vi "Lab Panel V5.22.vi"() -> ()   [LabVIEW 2013] (continued)
                n1766 = property on="SET LAB01-2" class="Clust (strict)"("DisabledEnum"=w3311) -> ()  [unwired: 2 in, 2 out]
                n1767 = property on="SET LAB02-1" class="Clust (strict)"("DisabledEnum"=w3310) -> ()  [unwired: 2 in, 2 out]
                n1768 = property on="SET LAB02-2" class="Clust (strict)"("DisabledEnum"=w3309) -> ()  [unwired: 2 in, 2 out]
                n1769 = property on="SET LAB03-1" class="Clust (strict)"("DisabledEnum"=w3308) -> ()  [unwired: 2 in, 2 out]
                n1770 = property on="O/I  LAB01-1" class="Bool (strict)"("DisabledEnum"=w3312) -> ()  [unwired: 2 in, 2 out]
                n1771 = property on="O/I  LAB01-2" class="Bool (strict)"("DisabledEnum"=w3311) -> ()  [unwired: 2 in, 2 out]
                n1772 = property on="O/I  LAB02-1" class="Bool (strict)"("DisabledEnum"=w3310) -> ()  [unwired: 2 in, 2 out]
                n1773 = property on="O/I  LAB02-2" class="Bool (strict)"("DisabledEnum"=w3309) -> ()  [unwired: 2 in, 2 out]
                n1774 = property on="O/I  LAB03-1" class="Bool (strict)"("DisabledEnum"=w3308) -> ()  [unwired: 2 in, 2 out]
              }
              frame #1 {
                n1775 = Select(t=2, s=w3342, f=0) -> (s? t:f=w3333:i32)
                n1776 = Select(t=2, s=w3341, f=0) -> (s? t:f=w3334:i32)
                n1777 = Select(t=2, s=w3338, f=0) -> (s? t:f=w3337:i32)
                n1778 = Select(t=2, s=w3339, f=0) -> (s? t:f=w3336:i32)
                n1779 = Select(t=2, s=w3340, f=0) -> (s? t:f=w3335:i32)
                n1780 = property on="SELECT LAB05-2" class="RadioBtnsControl (strict)"("DisabledEnum"=w3333) -> ()  [unwired: 2 in, 2 out]
                n1781 = property on="SELECT LAB05-1" class="RadioBtnsControl (strict)"("DisabledEnum"=w3334) -> ()  [unwired: 2 in, 2 out]
                n1782 = property on="SELECT LAB03-2" class="RadioBtnsControl (strict)"("DisabledEnum"=w3337) -> ()  [unwired: 2 in, 2 out]
                n1783 = property on="SELECT LAB04-1" class="RadioBtnsControl (strict)"("DisabledEnum"=w3336) -> ()  [unwired: 2 in, 2 out]
                n1784 = property on="SELECT LAB04-2" class="RadioBtnsControl (strict)"("DisabledEnum"=w3335) -> ()  [unwired: 2 in, 2 out]
                n1785 = property on="SET LAB05-2" class="Clust (strict)"("DisabledEnum"=w3333) -> ()  [unwired: 2 in, 2 out]
                n1786 = property on="SET LAB05-1" class="Clust (strict)"("DisabledEnum"=w3334) -> ()  [unwired: 2 in, 2 out]
                n1787 = property on="SET LAB03-2" class="Clust (strict)"("DisabledEnum"=w3337) -> ()  [unwired: 2 in, 2 out]
                n1788 = property on="SET LAB04-1" class="Clust (strict)"("DisabledEnum"=w3336) -> ()  [unwired: 2 in, 2 out]
                n1789 = property on="SET LAB04-2" class="Clust (strict)"("DisabledEnum"=w3335) -> ()  [unwired: 2 in, 2 out]
                n1790 = property on="O/I  LAB05-2" class="Bool (strict)"("DisabledEnum"=w3333) -> ()  [unwired: 2 in, 2 out]
                n1791 = property on="O/I  LAB05-1" class="Bool (strict)"("DisabledEnum"=w3334) -> ()  [unwired: 2 in, 2 out]
                n1792 = property on="O/I  LAB04-1" class="Bool (strict)"("DisabledEnum"=w3336) -> ()  [unwired: 2 in, 2 out]
                n1793 = property on="O/I  LAB04-2" class="Bool (strict)"("DisabledEnum"=w3335) -> ()  [unwired: 2 in, 2 out]
                n1794 = property on="O/I  LAB03-2" class="Bool (strict)"("DisabledEnum"=w3337) -> ()  [unwired: 2 in, 2 out]
                n1795 = Not(x=w3342) -> (.not. x?=w3343:bool)
                n1796 = Not(x=w3341) -> (.not. x?=w3344:bool)
                n1797 = Not(x=w3340) -> (.not. x?=w3345:bool)
                n1798 = property on="RESULT LAB05-2" class="Bool (strict)"("Visible"=w3343) -> ()  [unwired: 2 in, 2 out]
                n1799 = property on="RESULT LAB05-1" class="Bool (strict)"("Visible"=w3344) -> ()  [unwired: 2 in, 2 out]
                n1800 = Not(x=w3339) -> (.not. x?=w3346:bool)
                n1801 = property on="RESULT LAB04-2" class="Bool (strict)"("Visible"=w3345) -> ()  [unwired: 2 in, 2 out]
                n1802 = Not(x=w3338) -> (.not. x?=w3347:bool)
                n1803 = property on="RESULT LAB04-1" class="Bool (strict)"("Visible"=w3346) -> ()  [unwired: 2 in, 2 out]
                n1804 = property on="RESULT LAB03-2" class="Bool (strict)"("Visible"=w3347) -> ()  [unwired: 2 in, 2 out]
              }
              frame #2 {
                # "disable calibrate if any test running"
                n1805 = Or(x=w3370, y=w3369) -> (x .or. y?=w3363:bool)
                n1806 = Or(x=w3372, y=w3371) -> (x .or. y?=w3365:bool)
                n1807 = Or(x=w3376, y=w3375) -> (x .or. y?=w3367:bool)
                n1808 = Or(x=w3374, y=w3373) -> (x .or. y?=w3366:bool)
                n1809 = Or(x=w3378, y=w3377) -> (x .or. y?=w3368:bool)
                n1810 = Or(x=w3366, y=w3365) -> (x .or. y?=w3364:bool)
                n1811 = Or(x=w3368, y=w3367) -> (x .or. y?=w3362:bool)
                n1812 = Or(x=w3364, y=w3363) -> (x .or. y?=w3361:bool)
                n1813 = Or(x=w3362, y=w3361) -> (x .or. y?=w3360:bool)
                n1814 = case shown="False" w3360 {
                  tunnel: [0 2] -> w3359
                  frame False {
                  }
                  frame True {
                  }
                }
                n1815 = property on="JIG TEST" class="Clust (strict)"("DisabledEnum"=w3359) -> ()  [unwired: 2 in, 2 out]
                n1816 = property on="Network Directory" class="Path"("DisabledEnum"=w3359) -> ()  [unwired: 2 in, 2 out]
                n1817 = property on="MAIL SETTINGS" class="Clust (strict)"("DisabledEnum"=w3359) -> ()  [unwired: 2 in, 2 out]
                n1818 = property on="SET (cal)" class="Bool (strict)"("DisabledEnum"=w3359) -> ()  [unwired: 2 in, 2 out]
                n1819 = property on="ADMIN" class="Bool (strict)"("DisabledEnum"=0) -> ()  [unwired: 2 in, 2 out]
              }
            }
          }
          frame #8 {
            # "drive jigs"
            n1820 = stacked-sequence {
              frame #0 {
                # "jig on"
                n1821 = local read "jig cycle"() -> (w3386:dbl)
                n1822 = property on="JIG TEST" class="Clust (strict)"() -> ("DisabledEnum"=w3383:T16)  [unwired: 2 in, 2 out]
                n1823 = Equal?(x=w3383, y=2) -> (x = y?=w3382:bool)
                n1824 = Equal?(x=w3386, y=0) -> (x = y?=w3384:bool)
                n1825 = And(x=w3384, y=w3382) -> (x .and. y?=w3381:bool)
                n1826 = case shown="True" w3381 {
                  frame False {
                  }
                  frame True {
                    n1827 = local read "run lab01-1"() -> (w3397:bool)
                    n1828 = local read "run lab01-2"() -> (w3396:bool)
                    n1829 = local read "run lab02-1"() -> (w3395:bool)
                    n1830 = local read "run lab02-2"() -> (w3394:bool)
                    n1831 = local read "run lab03-1"() -> (w3393:bool)
                    n1832 = local read "run lab03-2"() -> (w3392:bool)
                    n1833 = local read "run lab04-1"() -> (w3391:bool)
                    n1834 = local read "run lab04-2"() -> (w3390:bool)
                    n1835 = local read "run lab05-1"() -> (w3389:bool)
                    n1836 = local read "run lab05-2"() -> (w3388:bool)
                    n1837 = local write "JIG LAB03-2"(w3392) -> ()
                    n1838 = local write "JIG LAB01-1"(w3397) -> ()
                    n1839 = local write "JIG LAB01-2"(w3396) -> ()
                    n1840 = local write "JIG LAB02-1"(w3395) -> ()
                    n1841 = local write "JIG LAB02-2"(w3394) -> ()
                    n1842 = local write "JIG LAB03-1"(w3393) -> ()
                    n1843 = local write "JIG LAB04-1"(w3391) -> ()
                    n1844 = local write "JIG LAB04-2"(w3390) -> ()
                    n1845 = local write "JIG LAB05-1"(w3389) -> ()
                    n1846 = local write "JIG LAB05-2"(w3388) -> ()
                  }
                }
              }
              frame #1 {
                # "jig off"
                n1847 = local read "jig cycle"() -> (w3404:dbl)
                n1848 = local read "on loops"() -> (w3403:dbl)
                n1849 = property on="JIG TEST" class="Clust (strict)"() -> ("DisabledEnum"=w3402:T16)  [unwired: 2 in, 2 out]
                n1850 = Equal?(x=w3402, y=2) -> (x = y?=w3400:bool)
                n1851 = Equal?(x=w3404, y=w3403) -> (x = y?=w3399:bool)
                n1852 = And(x=w3399, y=w3400) -> (x .and. y?=w3398:bool)
                n1853 = case shown="True" w3398 {
                  frame False {
                  }
                  frame True {
                    w3455 = FALSE
                    w3456 = TRUE
                    w3454 = 2
                    n1854 = local read "SELECT LAB05-2"() -> (w3445:T3)
                    n1855 = local read "SELECT LAB04-2"() -> (w3447:T3)
                    n1856 = local read "SELECT LAB04-1"() -> (w3448:T3)
                    n1857 = local read "SELECT LAB05-1"() -> (w3446:T3)
                    n1858 = local read "SELECT LAB03-2"() -> (w3449:T3)
                    n1859 = local read "SELECT LAB02-1"() -> (w3452:T3)
                    n1860 = local read "SELECT LAB03-1"() -> (w3450:T3)
                    n1861 = local read "SELECT LAB02-2"() -> (w3451:T3)
                    n1862 = local read "SELECT LAB01-2"() -> (w3453:T3)
                    n1863 = local read "run lab05-1"() -> (w3415:bool)
                    n1864 = local read "run lab05-2"() -> (w3414:bool)
                    n1865 = local read "SELECT LAB01-1"() -> (w3457:T3)
                    n1866 = local read "run lab04-2"() -> (w3416:bool)
                    n1867 = local read "run lab04-1"() -> (w3417:bool)
                    n1868 = local read "run lab01-1"() -> (w3433:bool)
                    n1869 = local read "run lab01-2"() -> (w3422:bool)
                    n1870 = local read "run lab03-2"() -> (w3418:bool)
                    n1871 = local read "run lab03-1"() -> (w3419:bool)
                    n1872 = local read "run lab02-1"() -> (w3421:bool)
                    n1873 = local read "run lab02-2"() -> (w3420:bool)
                    n1874 = Equal?(x=w3454, y=w3450) -> (x = y?=w3428:bool)
                    n1875 = Equal?(x=w3454, y=w3449) -> (x = y?=w3427:bool)
                    n1876 = Equal?(x=w3454, y=w3448) -> (x = y?=w3426:bool)
                    n1877 = Equal?(x=w3454, y=w3447) -> (x = y?=w3425:bool)
                    n1878 = Equal?(x=w3454, y=w3446) -> (x = y?=w3424:bool)
                    n1879 = Equal?(x=w3454, y=w3445) -> (x = y?=w3423:bool)
                    n1880 = Equal?(x=w3454, y=w3457) -> (x = y?=w3434:bool)
                    n1881 = Equal?(x=w3454, y=w3452) -> (x = y?=w3430:bool)
                    n1882 = Equal?(x=w3454, y=w3451) -> (x = y?=w3429:bool)
                    n1883 = Equal?(x=w3454, y=w3453) -> (x = y?=w3431:bool)
                    n1884 = And(x=w3425, y=w3416) -> (x .and. y?=w3407:bool)
                    n1885 = And(x=w3428, y=w3419) -> (x .and. y?=w3410:bool)
                    n1886 = And(x=w3426, y=w3417) -> (x .and. y?=w3408:bool)
                    n1887 = And(x=w3423, y=w3414) -> (x .and. y?=w3405:bool)
                    n1888 = And(x=w3429, y=w3420) -> (x .and. y?=w3411:bool)
                    n1889 = And(x=w3427, y=w3418) -> (x .and. y?=w3409:bool)
                    n1890 = And(x=w3424, y=w3415) -> (x .and. y?=w3406:bool)
                    n1891 = And(x=w3431, y=w3422) -> (x .and. y?=w3413:bool)
                    n1892 = And(x=w3434, y=w3433) -> (x .and. y?=w3432:bool)
                    n1893 = And(x=w3430, y=w3421) -> (x .and. y?=w3412:bool)
                    n1894 = Select(t=w3456, s=w3432, f=w3455) -> (s? t:f=w3435:bool)
                    n1895 = Select(t=w3456, s=w3413, f=w3455) -> (s? t:f=w3436:bool)
                    n1896 = Select(t=w3456, s=w3412, f=w3455) -> (s? t:f=w3437:bool)
                    n1897 = Select(t=w3456, s=w3411, f=w3455) -> (s? t:f=w3438:bool)
                    n1898 = Select(t=w3456, s=w3410, f=w3455) -> (s? t:f=w3439:bool)
                    n1899 = Select(t=w3456, s=w3409, f=w3455) -> (s? t:f=w3440:bool)
                    n1900 = Select(t=w3456, s=w3408, f=w3455) -> (s? t:f=w3441:bool)
                    n1901 = Select(t=w3456, s=w3407, f=w3455) -> (s? t:f=w3442:bool)
                    n1902 = Select(t=w3456, s=w3406, f=w3455) -> (s? t:f=w3443:bool)
                    n1903 = Select(t=w3456, s=w3405, f=w3455) -> (s? t:f=w3444:bool)
                    n1904 = local write "JIG LAB03-2"(w3440) -> ()
                    n1905 = local write "JIG LAB02-1"(w3437) -> ()
                    n1906 = local write "JIG LAB02-2"(w3438) -> ()
                    n1907 = local write "JIG LAB01-2"(w3436) -> ()
                    n1908 = local write "JIG LAB03-1"(w3439) -> ()
                    n1909 = local write "JIG LAB01-1"(w3435) -> ()
                    n1910 = local write "JIG LAB05-2"(w3444) -> ()
                    n1911 = local write "JIG LAB04-1"(w3441) -> ()
                    n1912 = local write "JIG LAB05-1"(w3443) -> ()
                    n1913 = local write "JIG LAB04-2"(w3442) -> ()
                  }
                }
              }
            }
          }
          frame #9 {
            # "enable  jig test output if no test busy"
            n1914 = property on="JIG TEST" class="Clust (strict)"() -> ("DisabledEnum"=w3460:T16)  [unwired: 2 in, 2 out]
            n1915 = Equal?(x=w3460, y=0) -> (x = y?=w3458:bool)
            n1916 = case shown="True" w3458 {
              frame False {
              }
              frame True {
                n1917 = local read "JIG TEST"() -> (w3471:T10)
                n1918 = Unbundle(w3471) -> ("LAB01-1"=w3470:bool, "LAB01-2"=w3469:bool, "LAB02-1"=w3468:bool, "LAB02-2"=w3467:bool, "LAB03-1"=w3466:bool, "LAB03-2"=w3465:bool, "LAB04-1"=w3464:bool, "LAB04-2"=w3463:bool, "LAB05-1"=w3462:bool, "LAB05-2"=w3461:bool)
                n1919 = local write "JIG LAB05-1"(w3462) -> ()
                n1920 = local write "JIG LAB05-2"(w3461) -> ()
                n1921 = local write "JIG LAB04-1"(w3464) -> ()
                n1922 = local write "JIG LAB04-2"(w3463) -> ()
                n1923 = local write "JIG LAB03-2"(w3465) -> ()
                n1924 = local write "JIG LAB01-1"(w3470) -> ()
                n1925 = local write "JIG LAB02-1"(w3468) -> ()
                n1926 = local write "JIG LAB03-1"(w3466) -> ()
                n1927 = local write "JIG LAB01-2"(w3469) -> ()
                n1928 = local write "JIG LAB02-2"(w3467) -> ()
              }
            }
          }
          frame #10 {
            # "Drive digital output and reset USB and temperature network if required."
            n1929 = global read "Global display 3.vi" "cycle O/F"() -> (w3481:bool)
            n1930 = local read "O/I  LAB05-2"() -> (w3474:bool)
            n1931 = local read "O/I  LAB05-1"() -> (w3476:bool)
            n1932 = local read "JIG LAB05-2"() -> (w3473:bool)
            n1933 = local read "O/I  LAB04-2"() -> (w3478:bool)
            n1934 = local read "JIG LAB05-1"() -> (w3475:bool)
            n1935 = local read "JIG LAB04-2"() -> (w3477:bool)
            n1936 = local read "O/I  LAB03-1"() -> (w3492:bool)
            n1937 = local read "O/I  LAB04-1"() -> (w3488:bool)
            n1938 = local read "O/I  LAB02-1"() -> (w3496:bool)
            n1939 = local read "O/I  LAB02-2"() -> (w3494:bool)
            n1940 = local read "O/I  LAB03-2"() -> (w3490:bool)
            n1941 = local read "JIG LAB04-1"() -> (w3487:bool)
            n1942 = local read "JIG LAB03-2"() -> (w3489:bool)
            n1943 = local read "O/I  LAB01-2"() -> (w3498:bool)
            n1944 = local read "JIG LAB02-1"() -> (w3495:bool)
            n1945 = local read "JIG LAB02-2"() -> (w3493:bool)
            n1946 = local read "JIG LAB03-1"() -> (w3491:bool)
            n1947 = local read "O/I  LAB01-1"() -> (w3500:bool)
            n1948 = local read "JIG LAB01-2"() -> (w3497:bool)
            n1949 = local read "JIG LAB01-1"() -> (w3499:bool)
            n1950 = case shown="False" w3481 {
              tunnel: [w3598 FALSE] -> w3480
              frame False {
                n1951 = local read "Analog error"() -> (w3597:bool)
                n1952 = local read "Reset Measuring"() -> (w3596:bool)
                n1953 = Or(x=w3596, y=w3597) -> (x .or. y?=w3598:bool)
              }
              frame True {
              }
            }
            n1954 = Build Array(w3493, w3492, w3491, w3490, w3489, w3488, w3487) -> (w3485:bool[])
            n1955 = Build Array(w3500, w3499, w3498, w3497, w3496, w3495, w3494) -> (w3486:bool[])
            n1956 = Build Array(w3478, w3477, w3476, w3475, w3474, w3473, FALSE) -> (w3484:bool[])
            n1957 = Not(x=w3481) -> (.not. x?=w3482:bool)
            n1958 = local read "Simulate"() -> (w3483:bool)
            n1959 = And(x=w3482, y=w3480) -> (x .and. y?=w3479:bool)
            n1960 = stacked-sequence {
              tunnel: w3486 -> [w3504 w3510]
              tunnel: w3485 -> [w3503 w3509]
              tunnel: w3484 -> [w3502 w3508]
              tunnel: w3483 -> [w3501 w3511]
              tunnel: w3479 -> [_ w3512]
              frame #0 {
                # "drive outputs for normal use"
                n1961 = case shown="False" w3501 {
                  tunnel: w3504 -> [w3507 _]
                  tunnel: w3503 -> [w3506 _]
                  tunnel: w3502 -> [w3505 _]
                  frame False {
                    n1962 = call "sub vi - Drive Relays All v6.vi"("Array #2"=w3505, "Array #1"=w3506, "Array #0"=w3507) -> ()  [unwired: 8 in, 1 out]
                  }
                  frame True {
                  }
                }
              }
              frame #1 {
                # "USB  reset routine"
                n1963 = case shown="True" w3512 {
                  tunnel: w3511 -> [_ w3516]
                  tunnel: w3510 -> [_ w3515]
                  tunnel: w3509 -> [_ w3514]
                  tunnel: w3508 -> [_ w3513]
                  frame False {
                  }
                  frame True {
                    n1964 = stacked-sequence {
                      seq-local: [w3518 _ _ _] -> [_ w3524 _ _]
                      tunnel: w3516 -> [_ w3528 _ _]
                      tunnel: w3515 -> [_ w3527 _ _]
                      tunnel: w3514 -> [_ w3526 _ _]
                      tunnel: w3513 -> [_ w3525 _ _]
                      frame #0 {
                        n1965 = case shown="False" "Auto Reset" {
                          tunnel: [w3521 FALSE] -> w3519
                          frame False {
                            n1966 = Two Button Dialog(message="System reset") -> (T button?=w3521:bool)  [unwired: 2 in]
                          }
                          frame True {
                          }
                        }
                        n1967 = local write "Tab Control 2"(5) -> ()
                        n1968 = Or(x="Auto Reset", y=w3519) -> (x .or. y?=w3518:bool)
                      }
                      frame #1 {
                        n1969 = disable-structure shown="Disabled" {
                          disable-tunnel: w3528 -> [w3533 _]
                          disable-tunnel: w3527 -> [w3532 _]
                          disable-tunnel: w3526 -> [w3531 _]
                          disable-tunnel: w3525 -> [w3530 _]
                          disable-tunnel: w3524 -> [w3529 _]
                          frame Disabled {
                            n1970 = case shown="True" w3529 {
                              tunnel: w3533 -> [_ w3539]
                              tunnel: w3532 -> [_ w3538]
                              tunnel: w3531 -> [_ w3537]
                              tunnel: w3530 -> [_ w3536]
                              frame False {
                              }
                              frame True {
                                n1971 = stacked-sequence {
                                tunnel: w3539 -> [_ w3557 _]
                                tunnel: bool[] [] -> [w3542 w3556 w3566]
                                tunnel: w3538 -> [_ _ w3565]
                                tunnel: w3537 -> [w3541 _ w3564]
                                tunnel: w3536 -> [w3540 _ w3563]
                                tunnel: 3000 -> [w3543 _ w3562]
                                frame #0 {
                                # "switch off test stations for system reset"
                                n1972 = stacked-sequence {
                                tunnel: w3543 -> [w3547 w3551 w3553]
                                tunnel: w3542 -> [w3546 w3550 w3554]
                                tunnel: w3541 -> [w3545 _ _]
                                tunnel: w3540 -> [w3544 w3549 _]
                                frame #0 {
                                # "drive 1st 7 inputs"
                                n1973 = call "sub vi - Drive Relays All v6.vi"("Array #2"=w3544, "Array #1"=w3545, "Array #0"=w3546) -> ()  [unwired: 8 in, 1 out]
                                n1974 = call "Message Display V1.vi"("Message"="Delay off LAB 01-1 to 02-1", "Delay mS"=w3547) -> ()  [unwired: 10 in]
                                }
                                frame #1 {
                                # "drive 2nd 7 inputs"
                                n1975 = call "sub vi - Drive Relays All v6.vi"("Array #2"=w3549, "Array #1"=w3550, "Array #0"=w3550) -> ()  [unwired: 8 in, 1 out]
                                n1976 = call "Message Display V1.vi"("Message"="Delay off LAB 02-2 to 04-1", "Delay mS"=w3551) -> ()  [unwired: 10 in]
                                }
                                frame #2 {
                                # "drive 3rd 7 inputs"
                                n1977 = call "sub vi - Drive Relays All v6.vi"("Array #2"=w3554, "Array #1"=w3554, "Array #0"=w3554) -> ()  [unwired: 8 in, 1 out]
                                n1978 = call "Message Display V1.vi"("Message"="Delay off LAB 04-2 to 05-2", "Delay mS"=w3553) -> ()  [unwired: 10 in]
                                }
                                }
                                }
                                frame #1 {
                                # "reset all usb modules"
                                n1979 = stacked-sequence {
                                tunnel: w3557 -> [_ w3561]
                                tunnel: w3556 -> [w3559 _]
                                frame #0 {
                                n1980 = call "sub vi - Drive Relays All v6.vi"("Array #2"=bool[] [FALSE, FALSE, FALSE, FALSE, FALSE, FALSE, TRUE], "Array #1"=w3559, "Array #0"=w3559) -> ()  [unwired: 8 in, 1 out]
                                }
                                frame #1 {
                                n1981 = call "Reset Meas v 4.vi"("simulate"=w3561) -> ("Reset Error"=→"Reset Error":bool)  [unwired: 10 in]
                                }
                                }
                                }
                                frame #2 {
                                # "switch test stations back on after reset"
                                n1982 = stacked-sequence {
                                tunnel: w3566 -> [w3570 w3573 _]
                                tunnel: w3565 -> [w3569 w3575 w3580]
                                tunnel: w3562 -> [w3568 w3571 w3577]
                                tunnel: w3564 -> [_ w3574 w3579]
                                tunnel: w3563 -> [_ _ w3576]
                                frame #0 {
                                # "drive 1st 7 inputs"
                                n1983 = call "sub vi - Drive Relays All v6.vi"("Array #2"=w3570, "Array #1"=w3570, "Array #0"=w3569) -> ()  [unwired: 8 in, 1 out]
                                n1984 = call "Message Display V1.vi"("Message"="Delay on LAB 01-1 to 02-1", "Delay mS"=w3568) -> ()  [unwired: 10 in]
                                }
                                frame #1 {
                                # "drive 1st & 2nd outputs"
                                n1985 = call "sub vi - Drive Relays All v6.vi"("Array #2"=w3573, "Array #1"=w3574, "Array #0"=w3575) -> ()  [unwired: 8 in, 1 out]
                                n1986 = call "Message Display V1.vi"("Message"="Delay on LAB 02-2 to 04-1", "Delay mS"=w3571) -> ()  [unwired: 10 in]
                                }
                                frame #2 {
                                n1987 = call "sub vi - Drive Relays All v6.vi"("Array #2"=w3576, "Array #1"=w3579, "Array #0"=w3580) -> ()  [unwired: 8 in, 1 out]
                                n1988 = call "Message Display V1.vi"("Message"="Delay on LAB 04-2 to 05-2", "Delay mS"=w3577) -> ()  [unwired: 10 in]
                                }
                                }
                                }
                                }
                              }
                            }
                          }
                          frame Enabled {
                          }
                        }
                      }
                      frame #2 {
                        w3585 = 0
                        w3586 = FALSE
                        # "set all back to zero"
                        n1989 = local read "Total USB resets"() -> (w3582:dbl)
                        n1990 = local read "Resets Done"() -> (w3584:dbl)
                        n1991 = local write "Reset Measuring"(w3586) -> ()
                        n1992 = local write "Analog error"(w3586) -> ()
                        n1993 = local write "Error USB #0"(w3586) -> ()
                        n1994 = local write "Error USB #1"(w3586) -> ()
                        n1995 = local write "Error USB #2"(w3586) -> ()
                        n1996 = local write "Er USB#0"(w3585) -> ()
                        n1997 = local write "Er USB#1"(w3585) -> ()
                        n1998 = local write "Er USB#2"(w3585) -> ()
                        n1999 = Increment(x=w3582) -> (x+1=w3581:dbl)
                        n2000 = Increment(x=w3584) -> (x+1=→"Resets Done":dbl)
                        n2001 = local write "Total USB resets"(w3581) -> ()
                      }
                      frame #3 {
                        # "mail reset value"
                        n2002 = disable-structure shown="Disabled" {
                          frame Disabled {
                            n2003 = local read "Total USB resets"() -> (w3592:dbl)
                            n2004 = local read "MAIL SETTINGS"() -> (w3588:T7)
                            n2005 = local read "Mail Test File To:"() -> (w3593:string)
                            n2006 = Number To Decimal String(number=w3592) -> (decimal integer string=w3590:string)  [unwired: 1 in]
                            n2007 = Unbundle(w3588) -> ("OUT SERVER ADDRESS"=w3595:string, "FROM ACCOUNT"=w3594:string)  [unwired: 5 out]
                            n2008 = Concatenate Strings("Total USB resets: ", w3590) -> (w3589:string)
                            n2009 = call "sub vi - send mail v5.vi"("TO:"=w3593, "subject"=w3589, "from"=w3594, "out going server"=w3595) -> ("error out"=w3587:errorcluster)  [unwired: 11 in]
                            n2010 = Bundle(cluster=w3588, "mail error"=w3587) -> ()  [unwired: 6 in, 1 out]
                          }
                          frame Enabled {
                          }
                        }
                      }
                    }
                  }
                }
              }
            }
          }
          frame #11 {
            # "get all analog values from USB devices"
            n2011 = local read "on loops"() -> (w3606:dbl)
            n2012 = local read "jig cycle"() -> (w3603:dbl)
            n2013 = Add(x=w3606, y=1) -> (x+y=w3604:dbl)
            n2014 = Equal?(x=w3603, y=1) -> (x = y?=w3600:bool)
            n2015 = Equal?(x=w3603, y=w3604) -> (x = y?=w3602:bool)
            n2016 = Or(x=w3600, y=w3602) -> (x .or. y?=w3601:bool)
            n2017 = global write "Global display 3.vi" "cycle O/F"(w3600) -> ()
            n2018 = case shown="True" w3601 {
              tunnel: w3600 -> [_ w3610]
              frame False {
              }
              frame True {
                n2019 = local read "Simulate"() -> (w3613:bool)
                n2020 = case shown="False" w3613 {
                  tunnel: [w3629 0.3 ("Analog loop time")] -> w3620
                  tunnel: [w3628 dynamicdata[] [] ("array GRAPH")] -> w3619
                  tunnel: [w3627 w3634] -> w3618
                  tunnel: [w3626 w3634] -> w3617
                  tunnel: [w3625 w3634] -> w3616
                  tunnel: [w3624 w3634] -> w3615
                  tunnel: [w3623 w3634] -> w3614
                  tunnel: w3610 -> [_ w3638]
                  tunnel: [w3622 "Ambient Volts"] -> w3609
                  tunnel: [w3621 bool[] []] -> w3608
                  frame False {
                    n2021 = call "sub vi - Read Analog All v9.3.vi"() -> ("Analog loop time"=w3629:dbl, "array GRAPH"=w3628:dynamicdata[], "LAB01"=w3627:T26, "LAB02"=w3626:T27, "LAB03"=w3625:T28, "LAB04"=w3624:T29, "deg C"=w3622:dbl, "USB Error"=w3621:bool[], "LAB05"=w3623:T30)  [unwired: 7 in]
                  }
                  frame True {
                    n2022 = local read "ON amps"() -> (w3632:dbl)
                    n2023 = local read "OFF amps"() -> (w3633:dbl)
                    n2024 = local read "VOLTS"() -> (w3636:dbl)
                    n2025 = local read "PF"() -> (w3635:dbl)
                    n2026 = Select(t=w3632, s=w3638, f=w3633) -> (s? t:f=w3637:dbl)
                    n2027 = Bundle("OFF amps"=w3637, "VOLTS"=w3636, "PF"=w3635, "OFF amps"=w3637, "VOLTS"=w3636, "PF"=w3635) -> (w3634:T31)  [unwired: 1 in]
                  }
                }
                n2028 = local read "Simulate"() -> (w3612:bool)
                n2029 = stacked-sequence {
                  seq-local: [w3643 _ _ _ _ _ _ _] -> [_ _ _ _ _ _ _ _]
                  seq-local: [w3642 _ _ _ _ _ _ _] -> [_ _ _ _ _ _ _ _]
                  seq-local: [w3641 _ _ _ _ _ _ _] -> [_ _ _ _ _ _ _ w3838]
                  tunnel: w3620 -> [_ w3696 _ _ _ _ _ _]
                  tunnel: w3619 -> [_ w3693 _ _ _ _ _ _]
                  tunnel: w3618 -> [_ _ w3723 _ _ _ _ _]
                  tunnel: w3617 -> [_ _ _ w3751 _ _ _ _]
                  tunnel: w3616 -> [_ _ _ _ w3779 _ _ _]
                  tunnel: w3615 -> [_ _ _ _ _ w3807 _ _]
                  tunnel: w3614 -> [_ _ _ _ _ _ w3835 _]
                  tunnel: w3612 -> [_ _ w3722 w3750 w3778 w3806 w3834 w3840]
                  tunnel: T14 {"1  (A) cal"=1.0, "1 (V) cal"=1.0, "1 (PF) cal"=1.0, "1 (TL) cal"=1.0, "1 (TN) cal"=1.0, "2 (A) cal"=1.0, "2 (V) cal"=1.0, "2 (PF) cal"=1.0, "2 (TL) cal"=1.0, "2 (TN) cal"=1.0} ("CAL LAB01") -> [_ _ w3721 w3749 w3777 w3805 w3833 _]
                  tunnel: w3609 -> [_ _ _ _ _ _ _ w3839]
                  tunnel: w3608 -> [w3646 _ _ _ _ _ _ _]
                  frame #0 {
                    n2030 = Index Array(array=w3646, index=2) -> (element=w3641:bool)
                    n2031 = Index Array(array=w3646, index=1) -> (element=w3642:bool)
                    n2032 = Index Array(array=w3646, index=0) -> (element=w3643:bool)
                    n2033 = local write "Error USB #2"(w3641) -> ()
                    n2034 = local write "Error USB #0"(w3643) -> ()
                    n2035 = local write "Error USB #1"(w3642) -> ()
                    n2036 = stacked-sequence {
                      tunnel: w3643 -> [w3650 _ _ _]
                      tunnel: w3642 -> [_ w3655 _ _]
                      tunnel: 0 -> [w3649 w3654 w3659 _]
                      tunnel: w3641 -> [_ _ w3660 _]
                      frame #0 {
                        n2037 = case shown="True" w3650 {
                          tunnel: w3649 -> [w3651 _]
                          frame False {
                            n2038 = local write "Er USB#0"(w3651) -> ()
                          }
                          frame True {
                            n2039 = local read "Er USB#0"() -> (w3653:dbl)
                            n2040 = Increment(x=w3653) -> (x+1=→"Er USB#0":dbl)
                          }
                        }
                      }
                      frame #1 {
                        n2041 = case shown="True" w3655 {
                          tunnel: w3654 -> [w3656 _]
                          frame False {
                            n2042 = local write "Er USB#1"(w3656) -> ()
                          }
                          frame True {
                            n2043 = local read "Er USB#1"() -> (w3658:dbl)
                            n2044 = Increment(x=w3658) -> (x+1=→"Er USB#1":dbl)
                          }
                        }
                      }
                      frame #2 {
                        n2045 = case shown="True" w3660 {
                          tunnel: w3659 -> [w3661 _]
                          frame False {
                            n2046 = local write "Er USB#2"(w3661) -> ()
                          }
                          frame True {
                            n2047 = local read "Er USB#2"() -> (w3663:dbl)
                            n2048 = Increment(x=w3663) -> (x+1=→"Er USB#2":dbl)
                          }
                        }
                      }
                      frame #3 {
                        w3669 = 5
                        n2049 = local read "Er USB#2"() -> (w3670:dbl)
                        n2050 = local read "Er USB#0"() -> (w3672:dbl)
                        n2051 = local read "Er USB#1"() -> (w3671:dbl)
                        n2052 = Greater Or Equal?(x=w3672, y=w3669) -> (x >= y?=w3667:bool)
                        n2053 = Greater Or Equal?(x=w3671, y=w3669) -> (x >= y?=w3666:bool)
                        n2054 = Greater Or Equal?(x=w3670, y=w3669) -> (x >= y?=w3665:bool)
                        n2055 = Or(x=w3667, y=w3666) -> (x .or. y?=w3668:bool)
                        n2056 = Or(x=w3668, y=w3665) -> (x .or. y?=→"Analog error":bool)
                      }
                    }
                  }
                  frame #1 {
                    # "display graph data on ADM page"
                    n2057 = local write "AI"(TRUE) -> ()
                    n2058 = global write "Global 1.vi" "RATE(Hz)"("RATE (Hz)") -> ()
                    n2059 = global write "Global 1.vi" "SAMPLES"("SAMPLES") -> ()
                    n2060 = Index Array(array=w3693, index=6) -> (element=→"LAB04-1 (GRAPH)":dynamicdata)
                    n2061 = Index Array(array=w3693, index=7) -> (element=→"LAB04-2 (GRAPH)":dynamicdata)
                    n2062 = Index Array(array=w3693, index=9) -> (element=→"LAB05-2 (GRAPH)":dynamicdata)
                    n2063 = Index Array(array=w3693, index=8) -> (element=→"LAB05-1 (GRAPH)":dynamicdata)
                    n2064 = Index Array(array=w3693, index=5) -> (element=→"LAB03-2 (GRAPH)":dynamicdata)
                    n2065 = Index Array(array=w3693, index=0) -> (element=→"LAB01-1 (GRAPH)":dynamicdata)
                    n2066 = Index Array(array=w3693, index=1) -> (element=→"LAB01-2 (GRAPH)":dynamicdata)
                    n2067 = Index Array(array=w3693, index=2) -> (element=→"LAB02-1 (GRAPH)":dynamicdata)
                    n2068 = Index Array(array=w3693, index=3) -> (element=→"LAB02-2 (GRAPH)":dynamicdata)
                    n2069 = Index Array(array=w3693, index=4) -> (element=→"LAB03-1 (GRAPH)":dynamicdata)
                    "AI loop time" <- w3696
                  }
                  frame #2 {
                    n2070 = case shown="False" w3722 {
                      tunnel: [w3724 w3725] -> w3720
                      tunnel: w3721 -> [_ w3725]
                      frame False {
                        n2071 = local read "CAL LAB01"() -> (w3724:T14)
                      }
                      frame True {
                      }
                    }
                    n2072 = Unbundle By Name(w3723) -> ("OFF amps"=w3719:dbl, "VOLTS"=w3718:dbl, "PF"=w3717:dbl, "OFF amps"=w3716:dbl, "VOLTS"=w3715:dbl, "PF"=w3714:dbl)
                    n2073 = Unbundle By Name(w3720) -> ("1  (A) cal"=w3713:dbl, "1 (V) cal"=w3712:dbl, "1 (PF) cal"=w3711:dbl, "2 (A) cal"=w3710:dbl, "2 (V) cal"=w3709:dbl, "2 (PF) cal"=w3708:dbl)  [unwired: 4 out]
                    n2074 = Multiply(x=w3719, y=w3713) -> (x*y=w3706:dbl)
                    n2075 = Multiply(x=w3718, y=w3712) -> (x*y=w3705:dbl)
                    n2076 = Multiply(x=w3717, y=w3711) -> (x*y=w3704:dbl)
                    n2077 = Multiply(x=w3716, y=w3710) -> (x*y=w3702:dbl)
                    n2078 = Multiply(x=w3715, y=w3709) -> (x*y=w3701:dbl)
                    n2079 = Multiply(x=w3714, y=w3708) -> (x*y=w3700:dbl)
                    n2080 = local read "SIG LAB01-1"() -> (w3707:T2)
                    n2081 = local read "SIG LAB01-2"() -> (w3703:T2)
                    n2082 = Bundle By Name(cluster=w3707, "AMPS"=w3706, "VOLTS"=w3705, "PF"=w3704) -> (w3699:T2)
                    n2083 = Bundle By Name(cluster=w3703, "AMPS"=w3702, "VOLTS"=w3701, "PF"=w3700) -> (w3698:T2)
                    n2084 = global write "Global display 1.vi" "SIG LAB01-2"(w3698) -> ()
                    n2085 = global write "Global display 1.vi" "SIG LAB01-1"(w3699) -> ()
                    n2086 = local write "SIG LAB01-2"(w3698) -> ()
                    n2087 = local write "SIG LAB01-1"(w3699) -> ()
                  }
                  frame #3 {
                    n2088 = Unbundle By Name(w3751) -> ("OFF amps"=w3747:dbl, "VOLTS"=w3746:dbl, "PF"=w3745:dbl, "OFF amps"=w3744:dbl, "VOLTS"=w3743:dbl, "PF"=w3742:dbl)
                    n2089 = case shown="True" w3750 {
                      tunnel: [w3752 w3753] -> w3748
                      tunnel: w3749 -> [_ w3753]
                      frame False {
                        n2090 = local read "CAL LAB02"() -> (w3752:T15)
                      }
                      frame True {
                      }
                    }
                    n2091 = Unbundle By Name(w3748) -> ("1  (A) cal"=w3741:dbl, "1 (V) cal"=w3740:dbl, "1 (PF) cal"=w3739:dbl, "2 (A) cal"=w3738:dbl, "2 (V) cal"=w3737:dbl, "2 (PF) cal"=w3736:dbl)  [unwired: 4 out]
                    n2092 = Multiply(x=w3747, y=w3741) -> (x*y=w3734:dbl)
                    n2093 = Multiply(x=w3746, y=w3740) -> (x*y=w3733:dbl)
                    n2094 = Multiply(x=w3745, y=w3739) -> (x*y=w3732:dbl)
                    n2095 = Multiply(x=w3744, y=w3738) -> (x*y=w3730:dbl)
                    n2096 = Multiply(x=w3743, y=w3737) -> (x*y=w3729:dbl)
                    n2097 = Multiply(x=w3742, y=w3736) -> (x*y=w3728:dbl)
                    n2098 = local read "SIG LAB02-1"() -> (w3735:T2)
                    n2099 = local read "SIG LAB02-2"() -> (w3731:T2)
                    n2100 = Bundle By Name(cluster=w3735, "AMPS"=w3734, "VOLTS"=w3733, "PF"=w3732) -> (w3727:T2)
                    n2101 = Bundle By Name(cluster=w3731, "AMPS"=w3730, "VOLTS"=w3729, "PF"=w3728) -> (w3726:T2)
                    n2102 = global write "Global display 1.vi" "SIG LAB02-1"(w3727) -> ()
                    n2103 = local write "SIG LAB02-2"(w3726) -> ()
                    n2104 = global write "Global display 1.vi" "SIG LAB02-2"(w3726) -> ()
                    n2105 = local write "SIG LAB02-1"(w3727) -> ()
                  }
                  frame #4 {
                    n2106 = Unbundle By Name(w3779) -> ("OFF amps"=w3775:dbl, "VOLTS"=w3774:dbl, "PF"=w3773:dbl, "OFF amps"=w3772:dbl, "VOLTS"=w3771:dbl, "PF"=w3770:dbl)
                    n2107 = case shown="True" w3778 {
                      tunnel: [w3780 w3781] -> w3776
                      tunnel: w3777 -> [_ w3781]
                      frame False {
                        n2108 = local read "CAL LAB03"() -> (w3780:T14)
                      }
                      frame True {
                      }
                    }
                    n2109 = Unbundle By Name(w3776) -> ("1  (A) cal"=w3769:dbl, "1 (V) cal"=w3768:dbl, "1 (PF) cal"=w3767:dbl, "2 (A) cal"=w3766:dbl, "2 (V) cal"=w3765:dbl, "2 (PF) cal"=w3764:dbl)  [unwired: 4 out]
                    n2110 = Multiply(x=w3775, y=w3769) -> (x*y=w3762:dbl)
                    n2111 = Multiply(x=w3774, y=w3768) -> (x*y=w3756:dbl)
                    n2112 = Multiply(x=w3773, y=w3767) -> (x*y=w3761:dbl)
                    n2113 = Multiply(x=w3772, y=w3766) -> (x*y=w3759:dbl)
                    n2114 = Multiply(x=w3771, y=w3765) -> (x*y=w3758:dbl)
                    n2115 = Multiply(x=w3770, y=w3764) -> (x*y=w3757:dbl)
                    n2116 = local read "SIG LAB03-1"() -> (w3763:T2)
                    n2117 = local read "SIG LAB03-2"() -> (w3760:T2)
                    n2118 = Bundle By Name(cluster=w3763, "AMPS"=w3762, "VOLTS"=w3756, "PF"=w3761) -> (w3755:T2)
                    n2119 = Bundle By Name(cluster=w3760, "AMPS"=w3759, "VOLTS"=w3758, "PF"=w3757) -> (w3754:T2)
                    n2120 = global write "Global display 1.vi" "SIG LAB03-1"(w3755) -> ()
                    n2121 = global write "Global display 1.vi" "SIG LAB03-2"(w3754) -> ()
                    n2122 = local write "SIG LAB03-2"(w3754) -> ()
                    n2123 = local write "SIG LAB03-1"(w3755) -> ()
                  }
                  frame #5 {
                    n2124 = case shown="False" w3806 {
                      tunnel: [w3808 w3809] -> w3804
                      tunnel: w3805 -> [_ w3809]
                      frame False {
                        n2125 = local read "CAL LAB04"() -> (w3808:T14)
                      }
                      frame True {
                      }
                    }
                    n2126 = Unbundle By Name(w3807) -> ("OFF amps"=w3803:dbl, "VOLTS"=w3802:dbl, "PF"=w3801:dbl, "OFF amps"=w3800:dbl, "VOLTS"=w3799:dbl, "PF"=w3798:dbl)
                    n2127 = Unbundle By Name(w3804) -> ("1  (A) cal"=w3797:dbl, "1 (V) cal"=w3796:dbl, "1 (PF) cal"=w3795:dbl, "2 (A) cal"=w3794:dbl, "2 (V) cal"=w3793:dbl, "2 (PF) cal"=w3792:dbl)  [unwired: 4 out]
                    n2128 = Multiply(x=w3803, y=w3797) -> (x*y=w3790:dbl)
                    n2129 = Multiply(x=w3802, y=w3796) -> (x*y=w3789:dbl)
                    n2130 = Multiply(x=w3801, y=w3795) -> (x*y=w3788:dbl)
                    n2131 = Multiply(x=w3800, y=w3794) -> (x*y=w3786:dbl)
                    n2132 = Multiply(x=w3799, y=w3793) -> (x*y=w3785:dbl)
                    n2133 = Multiply(x=w3798, y=w3792) -> (x*y=w3784:dbl)
                    n2134 = local read "SIG LAB04-1"() -> (w3791:T2)
                    n2135 = local read "SIG LAB04-2"() -> (w3787:T2)
                    n2136 = Bundle By Name(cluster=w3791, "AMPS"=w3790, "VOLTS"=w3789, "PF"=w3788) -> (w3783:T2)
                    n2137 = Bundle By Name(cluster=w3787, "AMPS"=w3786, "VOLTS"=w3785, "PF"=w3784) -> (w3782:T2)
                    n2138 = global write "Global display 1.vi" "SIG LAB04-2"(w3782) -> ()
                    n2139 = global write "Global display 1.vi" "SIG LAB04-1"(w3783) -> ()
                    n2140 = local write "SIG LAB04-2"(w3782) -> ()
                    n2141 = local write "SIG LAB04-1"(w3783) -> ()
                  }
                  frame #6 {
                    n2142 = Unbundle By Name(w3835) -> ("OFF amps"=w3831:dbl, "VOLTS"=w3812:dbl, "PF"=w3830:dbl, "OFF amps"=w3829:dbl, "VOLTS"=w3828:dbl, "PF"=w3827:dbl)
                    n2143 = case shown="False" w3834 {
                      tunnel: [w3836 w3837] -> w3832
                      tunnel: w3833 -> [_ w3837]
                      frame False {
                        n2144 = local read "CAL LAB05"() -> (w3836:T14)
                      }
                      frame True {
                      }
                    }
                    n2145 = Unbundle By Name(w3832) -> ("1  (A) cal"=w3826:dbl, "1 (V) cal"=w3825:dbl, "1 (PF) cal"=w3824:dbl, "2 (A) cal"=w3823:dbl, "2 (V) cal"=w3822:dbl, "2 (PF) cal"=w3821:dbl)  [unwired: 4 out]
                    n2146 = Multiply(x=w3831, y=w3826) -> (x*y=w3819:dbl)
                    n2147 = Multiply(x=w3812, y=w3825) -> (x*y=w3818:dbl)
                    n2148 = Multiply(x=w3830, y=w3824) -> (x*y=w3817:dbl)
                    n2149 = Multiply(x=w3829, y=w3823) -> (x*y=w3815:dbl)
                    n2150 = Multiply(x=w3828, y=w3822) -> (x*y=w3814:dbl)
                    n2151 = Multiply(x=w3827, y=w3821) -> (x*y=w3813:dbl)
                    n2152 = local read "SIG LAB05-1"() -> (w3820:T2)
                    n2153 = local read "SIG LAB05-2"() -> (w3816:T2)
                    n2154 = Bundle By Name(cluster=w3820, "AMPS"=w3819, "VOLTS"=w3818, "PF"=w3817) -> (w3811:T2)
                    n2155 = Bundle By Name(cluster=w3816, "AMPS"=w3815, "VOLTS"=w3814, "PF"=w3813) -> (w3810:T2)
                    n2156 = global write "Global display 1.vi" "SIG LAB05-1"(w3811) -> ()
                    n2157 = global write "Global display 1.vi" "SIG LAB05-2"(w3810) -> ()
                    n2158 = local write "SIG LAB05-2"(w3810) -> ()
                    n2159 = local write "SIG LAB05-1"(w3811) -> ()
                  }
                  frame #7 {
                    n2160 = case shown="False" w3838 {
                      tunnel: w3840 -> [w3842 _]
                      tunnel: w3839 -> [w3841 _]
                      frame False {
                        # "update ambient referance temperature"
                        n2161 = case shown="True" w3842 {
                          tunnel: [w3845 100.0] -> w3844
                          frame False {
                            n2162 = local read "TEMP REF cal"() -> (w3845:dbl)
                          }
                          frame True {
                          }
                        }
                        n2163 = local read "Panel #"() -> (w3843:dbl)
                        n2164 = case shown="1" w3843 {
                          tunnel: w3844 -> [_ w3851]
                          tunnel: w3841 -> [_ w3850]
                          frame 0, Default {
                          }
                          frame 1 {
                            n2165 = Multiply(x=w3851, y=w3850) -> (x*y=w3849:dbl)
                            n2166 = Subtract(x=w3849, y=272) -> (x-y=w3847:dbl)
                            "Amb Tp" <- w3847
                            n2167 = local write "Ref deg C"(w3847) -> ()
                          }
                        }
                        "deg C (volts)" <- w3841
                      }
                      frame True {
                      }
                    }
                  }
                }
              }
            }
          }
          frame #12 {
            # "save test data to file"
            n2168 = Get Date/Time In Seconds() -> (seconds since 1Jan1904=w3852:timestamp)
            "File Time Stamp" <- w3852
            n2169 = local read "on loops"() -> (w3871:dbl)
            n2170 = local read "jig cycle"() -> (w3868:dbl)
            n2171 = Format Date/Time String(time format string (%c)="%H:%M%:%S", seconds (now)=w3852) -> (date/time string=w3856:string)  [unwired: 1 in]
            n2172 = Add(x=w3871, y=2) -> (x+y=w3869:dbl)
            n2173 = Build Array(w3856) -> (w3855:string[])
            n2174 = Equal?(x=w3868, y=1) -> (x = y?=w3854:bool)
            n2175 = Equal?(x=w3868, y=w3869) -> (x = y?=w3853:bool)
            n2176 = stacked-sequence {
              tunnel: w3867 -> [w3877 _ _ _ _ _ _ _ _ _]
              tunnel: w3866 -> [_ w3953 _ _ _ _ _ _ _ _]
              tunnel: w3865 -> [_ _ w4033 _ _ _ _ _ _ _]
              tunnel: w3864 -> [_ _ _ w4113 _ _ _ _ _ _]
              tunnel: w3863 -> [_ _ _ _ w4193 _ _ _ _ _]
              tunnel: w3862 -> [_ _ _ _ _ w4273 _ _ _ _]
              tunnel: w3861 -> [_ _ _ _ _ _ w4353 _ _ _]
              tunnel: w3860 -> [_ _ _ _ _ _ _ w4433 _ _]
              tunnel: w3859 -> [_ _ _ _ _ _ _ _ w4513 _]
              tunnel: w3858 -> [_ _ _ _ _ _ _ _ _ w4593]
              tunnel: w3855 -> [w3876 w3957 w4037 w4117 w4197 w4277 w4357 w4437 w4517 w4597]
              tunnel: w3854 -> [w3875 w3956 w4036 w4116 w4196 w4276 w4356 w4436 w4516 w4596]
              tunnel: w3853 -> [w3874 w3955 w4035 w4115 w4195 w4275 w4355 w4435 w4515 w4595]
              tunnel: w3852 -> [w3873 w3954 w4034 w4114 w4194 w4274 w4354 w4434 w4514 w4594]
              frame #0 {
                n2177 = case shown="True" w3877 {
                  tunnel: w3876 -> [_ w3882]
                  tunnel: w3875 -> [_ w3881]
                  tunnel: w3874 -> [_ w3879]
                  tunnel: w3873 -> [_ w3878]
                  frame False {
                  }
                  frame True {
                    n2178 = local read "DISP LAB01-1"() -> (w3883:T4)
                    n2179 = local read "SIG LAB01-1"() -> (w3884:T2)
                    n2180 = local read "ON L01-1"() -> (w3880:cluster{"amps":dbl, "volts":dbl, "pf":dbl})
                    n2181 = Unbundle(w3884) -> ("AMPS"=w3890:dbl, "VOLTS"=w3888:dbl, "PF"=w3887:dbl, "Tmp Live"=w3886:dbl, "Tmp Neut"=w3889:dbl)
                    n2182 = Unbundle(w3883) -> ("CYCLE"=w3885:dbl)  [unwired: 2 out]
                    n2183 = stacked-sequence {
                      tunnel: w3890 -> [w3894 w3913]
                      tunnel: w3889 -> [_ w3912]
                      tunnel: w3888 -> [w3893 w3911]
                      tunnel: w3887 -> [w3892 w3910]
                      tunnel: w3886 -> [_ w3909]
                      tunnel: w3885 -> [_ w3908]
                      tunnel: w3882 -> [_ w3907]
                      tunnel: w3881 -> [w3895 _]
                      tunnel: w3880 -> [w3891 w3905]
                      tunnel: w3879 -> [_ w3906]
                      tunnel: w3878 -> [_ w3901]
